vi "JSON string to cluster.vi"(11 "JSON status":string) -> (3 "Focuser160":T1)   [LabVIEW 2012]
panel:
  out "size(s)":i32
  out "array":string[](array[string])
  out "keywords":string[](array[string])
  # "{\n\"absolute\": true,\n\"alarm\": false,\n\"cmd\": {\n    \"clientId\": 1234,\n    \"clientTransactionId\": 9876,\n     \"clientName\": \"Focuser160\",\n     \"action\": \"MOVE=10\"\n     },\n\"connected\": true,\n\"controller\": \"Focuser160\",\n\"device\": \"Mirror2\",\n\"error\": \"\",\n\"homing\": false,\n\"initialized\": true,\n\"isMoving\": false,\n\"maxSpeed\": 150,\n\"maxStep\": 1000000,\n\"position\": 1549,\n\"tempComp\": false,\n\"tempCompAvailable\": false,\n“temperature”: 22,\n\"timestamp\": 1642577702.123\n}"
  # "O nome e o tipo de dados dos\ncontroles do indicador \"JSON cluster\" devem ser iguais aos \nkeywords e valores da string \"JSON status\"."
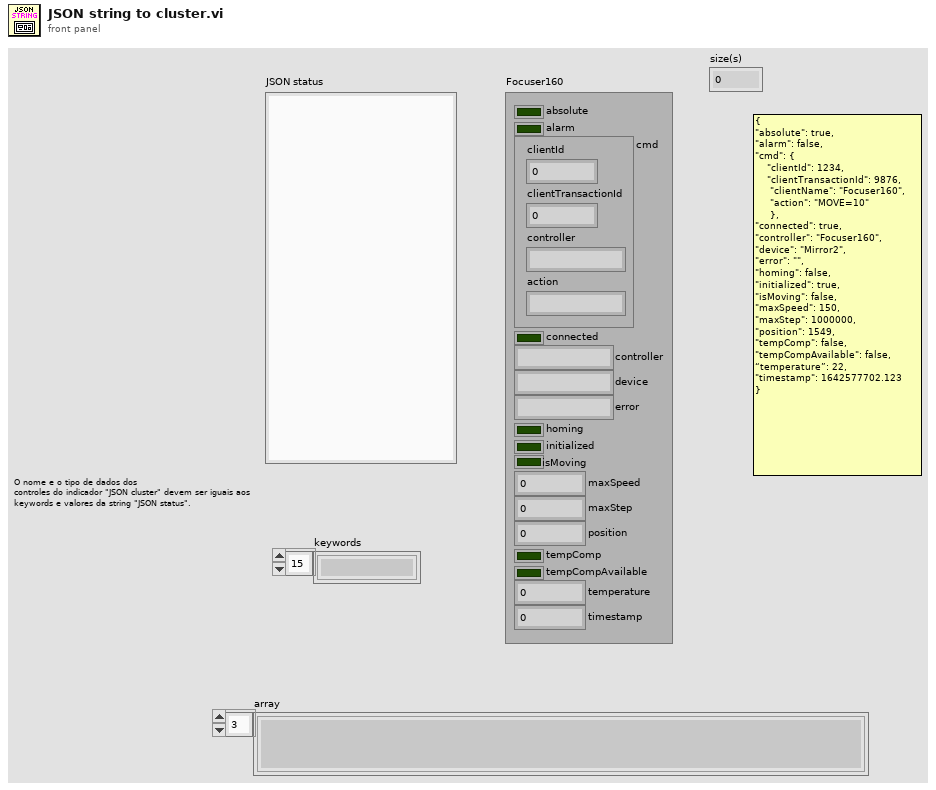
[diagram p1: front panel]
types:
  T1 = cluster{"absolute":bool, "alarm":bool, "cmd":cluster{"clientId":dbl, "clientTransactionId":dbl, "controller":string, "action":string}, "connected":bool, "controller":string, "device":string, "error":string, "homing":bool, "initialized":bool, "isMoving":bool, "maxSpeed":dbl, "maxStep":dbl, "position":dbl, "tempComp":bool, "tempCompAvailable":bool, "temperature":dbl, "timestamp":dbl}
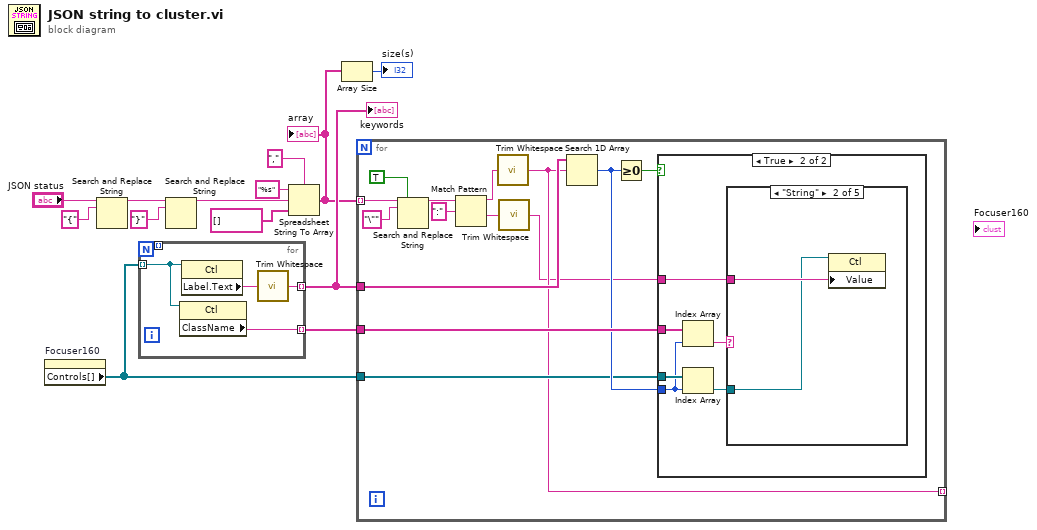
[diagram p0: block diagram]
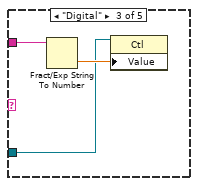
[diagram p4: hidden frame]
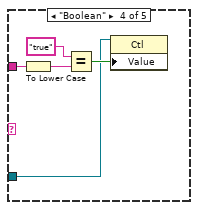
[diagram p5: hidden frame]
diagram:
  n1 = property on="Focuser160" class="Clust (strict)"() -> ("Controls[]"=w1:refnum<vi>[])  [unwired: 2 in, 2 out]
  n2 = Search and Replace String(input string="JSON status", search string="{") -> (result string=w5:string)  [unwired: 6 in, 3 out]
  n3 = for {
    N -> [w14]
    tunnel: w1 -> [w17] mode=indexing
    tunnel: [w15] -> w9 mode=indexing
    tunnel: [w16] -> w10 mode=indexing
    tunnel: [w14] -> _ mode=indexing
    n4 = property class="Ctl"(reference=w17) -> ("ClassName"=w16:string)  [unwired: 1 in, 2 out]
    n5 = property class="Ctl"(reference=w17) -> ("Label.Text"=w18:string)  [unwired: 1 in, 2 out]
    n6 = call <vilib>:"Trim Whitespace.vi"("string"=w18) -> ("trimmed string"=w15:string)  [unwired: 1 in]
  }
  "keywords" <- w9
  n7 = Search and Replace String(input string=w5, search string="}") -> (result string=w4:string)  [unwired: 6 in, 3 out]
  n8 = Spreadsheet String To Array(delimiter (Tab)=",", format string="%s", spreadsheet string=w4, array type (2D Dbl)=string[] [] ("Array 2")) -> (array=w3:string[])
  "array" <- w3
  n9 = Array Size(array=w3) -> (size(s)=→"size(s)":i32)
  n10 = for {
    tunnel: w3 -> [w21] mode=indexing
    tunnel: w9 -> [w29]
    tunnel: w10 -> [w26]
    tunnel: w1 -> [w24]
    tunnel: [w23] -> _ mode=indexing
    n11 = Search and Replace String(replace all?=TRUE ("replace all? (F)"), input string=w21, search string="\"") -> (result string=w20:string)  [unwired: 5 in, 3 out]
    n12 = Match Pattern(string=w20, regular expression=":") -> (before substring=w19:string, after substring=w27:string)  [unwired: 1 in, 2 out]
    n13 = call <vilib>:"Trim Whitespace.vi"("string"=w19) -> ("trimmed string"=w23:string)  [unwired: 1 in]
    n14 = call <vilib>:"Trim Whitespace.vi"("string"=w27) -> ("trimmed string"=w22:string)  [unwired: 1 in]
    n15 = Search 1D Array(1D array=w29, element=w23) -> (index of element=w25:i32)  [unwired: 1 in]
    n16 = Greater Or Equal To 0?(x=w25) -> (x >= 0?=w28:bool)
    n17 = case shown="True" w28 {
      tunnel: w22 -> [_ w36]
      tunnel: w26 -> [_ w38]
      tunnel: w25 -> [_ w34]
      tunnel: w24 -> [_ w35]
      frame False {
      }
      frame True {
        n18 = Index Array(array=w38, index=w34) -> (element=w37:string)
        n19 = Index Array(array=w35, index=w34) -> (element=w33:refnum<vi>)
        n20 = case shown="\"String\"" w37 {
          tunnel: w36 -> [_ w40 w43 w48 _]
          tunnel: w33 -> [_ w39 w41 w44 _]
          frame "NaN", Default {
          }
          frame "String" {
            n21 = property class="Ctl"(reference=w39, "Value"=w40) -> ()  [unwired: 1 in, 2 out]
          }
          frame "Digital" {
            n22 = Fract/Exp String To Number(string=w43) -> (number=w42:dbl)  [unwired: 3 in, 1 out]
            n23 = property class="Ctl"(reference=w41, "Value"=w42) -> ()  [unwired: 1 in, 2 out]
          }
          frame "Boolean" {
            n24 = To Lower Case(string=w48) -> (all lower case string=w46:string)
            n25 = Equal?(x="true", y=w46) -> (x = y?=w45:bool)
            n26 = property class="Ctl"(reference=w44, "Value"=w45) -> ()  [unwired: 1 in, 2 out]
          }
          frame "Cluster" {
          }
        }
      }
    }
  }
